vi "Read Enum U8.vi"(8 "error in (no error)":errorcluster, 11 "Numeric Types in":refnum<class "Numeric Types.lvclass">) -> (0 "error out":errorcluster, 2 "Enum U8":enum8{"One", "Two", "Three"}(ring), 3 "Numeric Types out":refnum<class "Numeric Types.lvclass">)   [LabVIEW 2017, in "Generic Object Serializer Tests.lvlib" / "Numeric Types.lvclass"]
uses:
  Numeric Types.lvclass
  Numeric Types.lvclass/Numeric Types.ctl
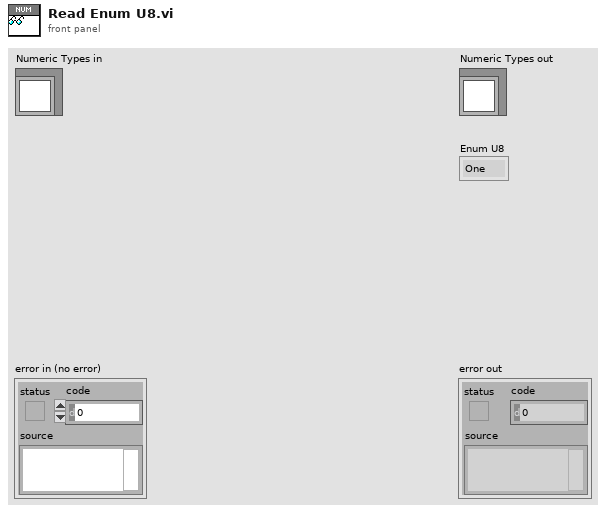
[diagram p1: front panel]
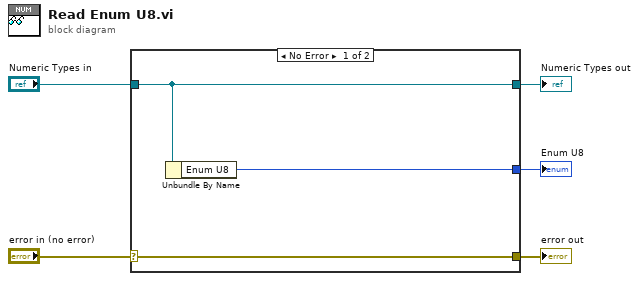
[diagram p0: block diagram]
diagram:
  n1 = case shown="No Error" "error in (no error)" {
    selector: "error in (no error)" -> [w8 w9]
    tunnel: [w8 w9] -> w4
    tunnel: [w7 w10] -> w2
    tunnel: "Numeric Types in" -> [w7 w10]
    tunnel: [w6 _] -> w1
    frame No Error {
      n2 = Unbundle By Name(w7) -> ("Enum U8"=w6:enum8{"One", "Two", "Three"})
    }
    frame Error {
    }
  }
  "error out" <- w4
  "Numeric Types out" <- w2
  "Enum U8" <- w1
